vi "waitForFirstImage.vi"(8 "error in (no error)":errorcluster, 9 "timeout_s":dbl=nan, 10 "delay":bool=TRUE, 11 "Camera in":refnum<class "Camera.lvclass">) -> (0 "error out":errorcluster, 3 "Camera out":refnum<class "Camera.lvclass">)   [LabVIEW 2019, in "Camera.lvclass"]
doc: "Waits for the first available image in the recorder memory. In recorder mode 'sequence non\nblocking', 'ring buffer'. and 'fifo', the function record.vi returns immediately.\nTherefore, this function can be used to wait for images from the camera before calling\nimage.vi, images.vi, or image_average.vi."
uses:
  Camera.lvclass
  Camera.lvclass/Camera.ctl
  pco.recorder/Recorder.lvlib
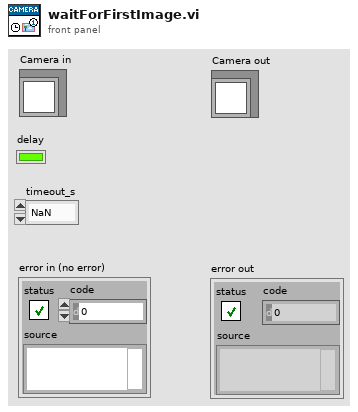
[diagram p1: front panel]
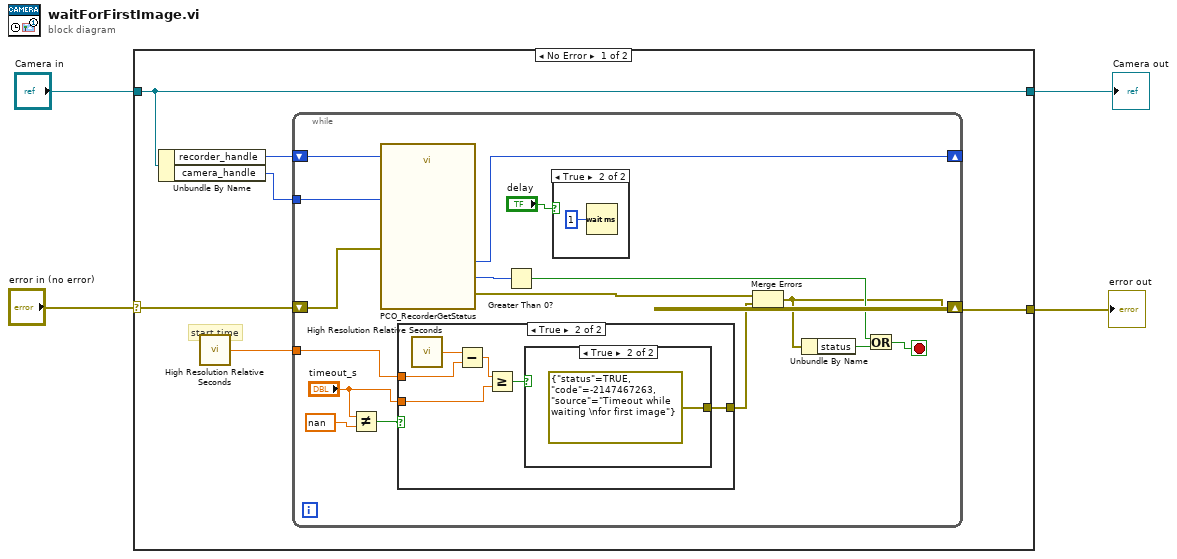
[diagram p0: block diagram]
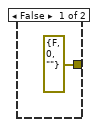
[diagram p2: hidden frame]
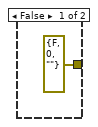
[diagram p3: hidden frame]
diagram:
  n1 = case shown="No Error" "error in (no error)" {
    selector: "error in (no error)" -> [w8 w38]
    tunnel: [w6 w38] -> w3
    tunnel: [w10 w37] -> w1
    tunnel: "Camera in" -> [w10 w37]
    frame No Error {
      # "start time"
      n2 = Unbundle By Name(w10) -> ("recorder_handle"=w9:u64, "camera_handle"=w7:u64)
      n3 = call <vilib>:"High Resolution Relative Seconds.vi"() -> ("relative seconds"=w5:dbl)
      n4 = while {
        shift-right: [w11] -> w6
        shift-left: w8 -> [w25]
        shift-right: [w24] -> _
        shift-left: w9 -> [w26]
        tunnel: w7 -> [w23]
        tunnel: w5 -> [w15]
        stop <- w19 stop-if-true
        n5 = Not Equal?(x="timeout_s", y=nan) -> (x != y?=w16:bool)
        n6 = call "PCO_RecorderGetStatus.vi"("phRec"=w26, "phCam"=w23, "error in (no error)"=w25) -> ("dwProcImgCount"=w22:u32, "phRec out"=w24:u64, "error out"=w12:errorcluster)  [unwired: 5 in, 9 out]
        n7 = case shown="True" w16 {
          tunnel: w15 -> [_ w32]
          tunnel: "timeout_s" -> [_ w30]
          tunnel: [errorcluster {"status"=FALSE, "code"=0, "source"=""} ("error constant") w28] -> w13
          frame False {
          }
          frame True {
            n8 = call <vilib>:"High Resolution Relative Seconds.vi"() -> ("relative seconds"=w33:dbl)
            n9 = Subtract(x=w33, y=w32) -> (x-y=w31:dbl)
            n10 = Greater Or Equal?(x=w31, y=w30) -> (x >= y?=w29:bool)
            n11 = case shown="True" w29 {
              tunnel: [errorcluster {"status"=FALSE, "code"=0, "source"=""} ("error constant") errorcluster {"status"=TRUE, "code"=-2147467263, "source"="Timeout while waiting \nfor first image"} ("error constant")] -> w28
              frame False {
              }
              frame True {
              }
            }
          }
        }
        n12 = Greater Than 0?(x=w22) -> (x > 0?=w20:bool)
        n13 = case shown="True" "delay" {
          frame False {
          }
          frame True {
            n14 = Wait (ms)(milliseconds to wait=u32 1) -> ()  [unwired: 1 out]
          }
        }
        n15 = Merge Errors(w12, w13) -> (w11:errorcluster)
        n16 = Unbundle By Name(w11) -> ("status"=w21:bool)
        n17 = Or(x=w20, y=w21) -> (x .or. y?=w19:bool)
      }
    }
    frame Error {
    }
  }
  "error out" <- w3
  "Camera out" <- w1
